vi "Main.vi"() -> ()   [LabVIEW 2020]
doc: "Use this template to build a simple state machine design pattern. Each state executes code and determines which state to transition to."
uses:
  Trigger Cluster.ctl
  TrigSource.ctl
  TrigLevel.ctl
  TrigSpeedCluster.ctl
  controls/State.ctl
  controls/Data.ctl
  MuessageCluster.ctl
  <vilib>/Utility/miscctls.llb/LVRangeTypeDef.ctl
  <vilib>/Utility/sysdir.llb/System Directory Type.ctl
  <vilib>/DAQmx/read.llb/DAQmx Read (Analog 1D Wfm NChan NSamp).vi
  <vilib>/DAQmx/read.llb/DAQmx Read (Counter 2D DBL NChan NSamp).vi
  <vilib>/DAQmx/miscellaneous.llb/DAQmx Fill In Error Info.vi
  <vilib>/measure/mamon.llb/Trigger Detection for 1 Channel.vi
  <vilib>/measure/NI_MAPro.lvlib
panel:
  in  "ManualTrigger":bool caption="Manual Record"
  in  "TrigSpeeds":T1 caption="Record Start/Stop Speeds" {"EndSpeed" min=0 max=12 step=0.1 format="%.1g"; "StartSpeed" min=0 max=12 step=0.1 format="%.1g"}
  in  "TrigCluster":T2={"TrigSource"=enum."Stop Key", "TrigLevel"=enum."Falling"} caption="Trigger Settings"
  out "Loop Time":i32
  out "StopButton":bool
  out "Recording":bool
  out "Trigger":bool
  out "PreTrigger":bool
  out "MPH":dbl format="%.1g"
  in  "Header Row Title":string
  out "Speed Chart":dbl(graph)
  in  "Exit":bool
  # "Treadmill Speed"
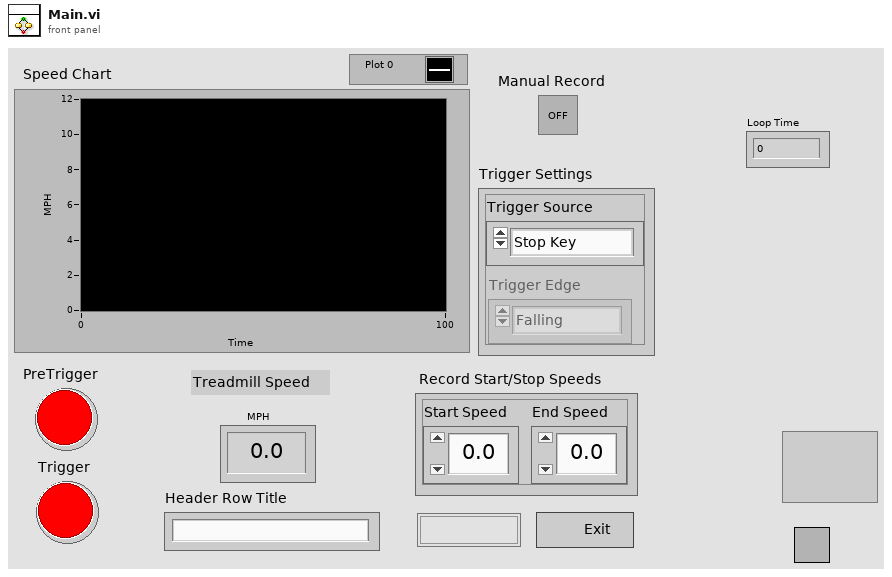
[diagram p1: front panel]
types:
  T1 = typedef "TrigSpeedCluster.ctl" = cluster{"StartSpeed":sgl, "EndSpeed":sgl}
  T2 = typedef "Trigger Cluster.ctl" = cluster{"TrigSource":T3, "TrigLevel":T4}
  T3 = typedef "TrigSource.ctl" = enum16{"Error Condition", "Machine Ctrl (Phase C)", "E-Stop Key", "Stop Key", "Blackout", "Manual"}
  T4 = typedef "TrigLevel.ctl" = enum16{"Falling", "Rising"}
  T5 = typedef "MuessageCluster.ctl" = cluster{"Message":enum16{"Init", "StopRFQ", "Stop", "UserEvent"}, "Message Data":variant}
  T6 = typedef "Data.ctl" = cluster{"Speed Data":dbl, "StopButtonState":bool, "Recording":bool, "PreTrigStateCount":u32, "HeaderString":string, "SpeedTask":refnum<k21>, "AnalogTrigTask":refnum<k21>, "TriggerLevel Data":waveform(dbl)[], "PreTrigTimer(s)":dbl, "MillisecondTimerValue":dbl, "RecordedData":dbl[][], "StopButton":bool, "TrigCluster":T2, "PreTrigState":bool, "TriggerState":bool, "TrigTimeStamp":dbl[], "TrigSpeeds":T1, "ResetTrig?":bool, "SpeedData":dbl[][], "ManualTrigger":bool}
  T7 = typedef "State.ctl" = enum16{"Initialize", "Start Tasks", "Acquire", "Check Trigger", "Check TriggerOrg", "Check for User Event", "StopRFQ", "Update UI", "CheckPreTrigState", "CheckPreTrigStateOrg", "Save MPH/Time Data", "Save Data to CSV", "Restart", "StreamingData", "Exit"}
  T8 = enum8{"Enabled", "Disabled", "Disabled and Grayed Out"}
  T9 = typedef "LVRangeTypeDef.ctl" = cluster{"Minimum":dbl, "Maximum":dbl, "Increment":dbl, "Minor Increment":dbl, "Start":dbl}
  T10 = typedef "System Directory Type.ctl" = i32
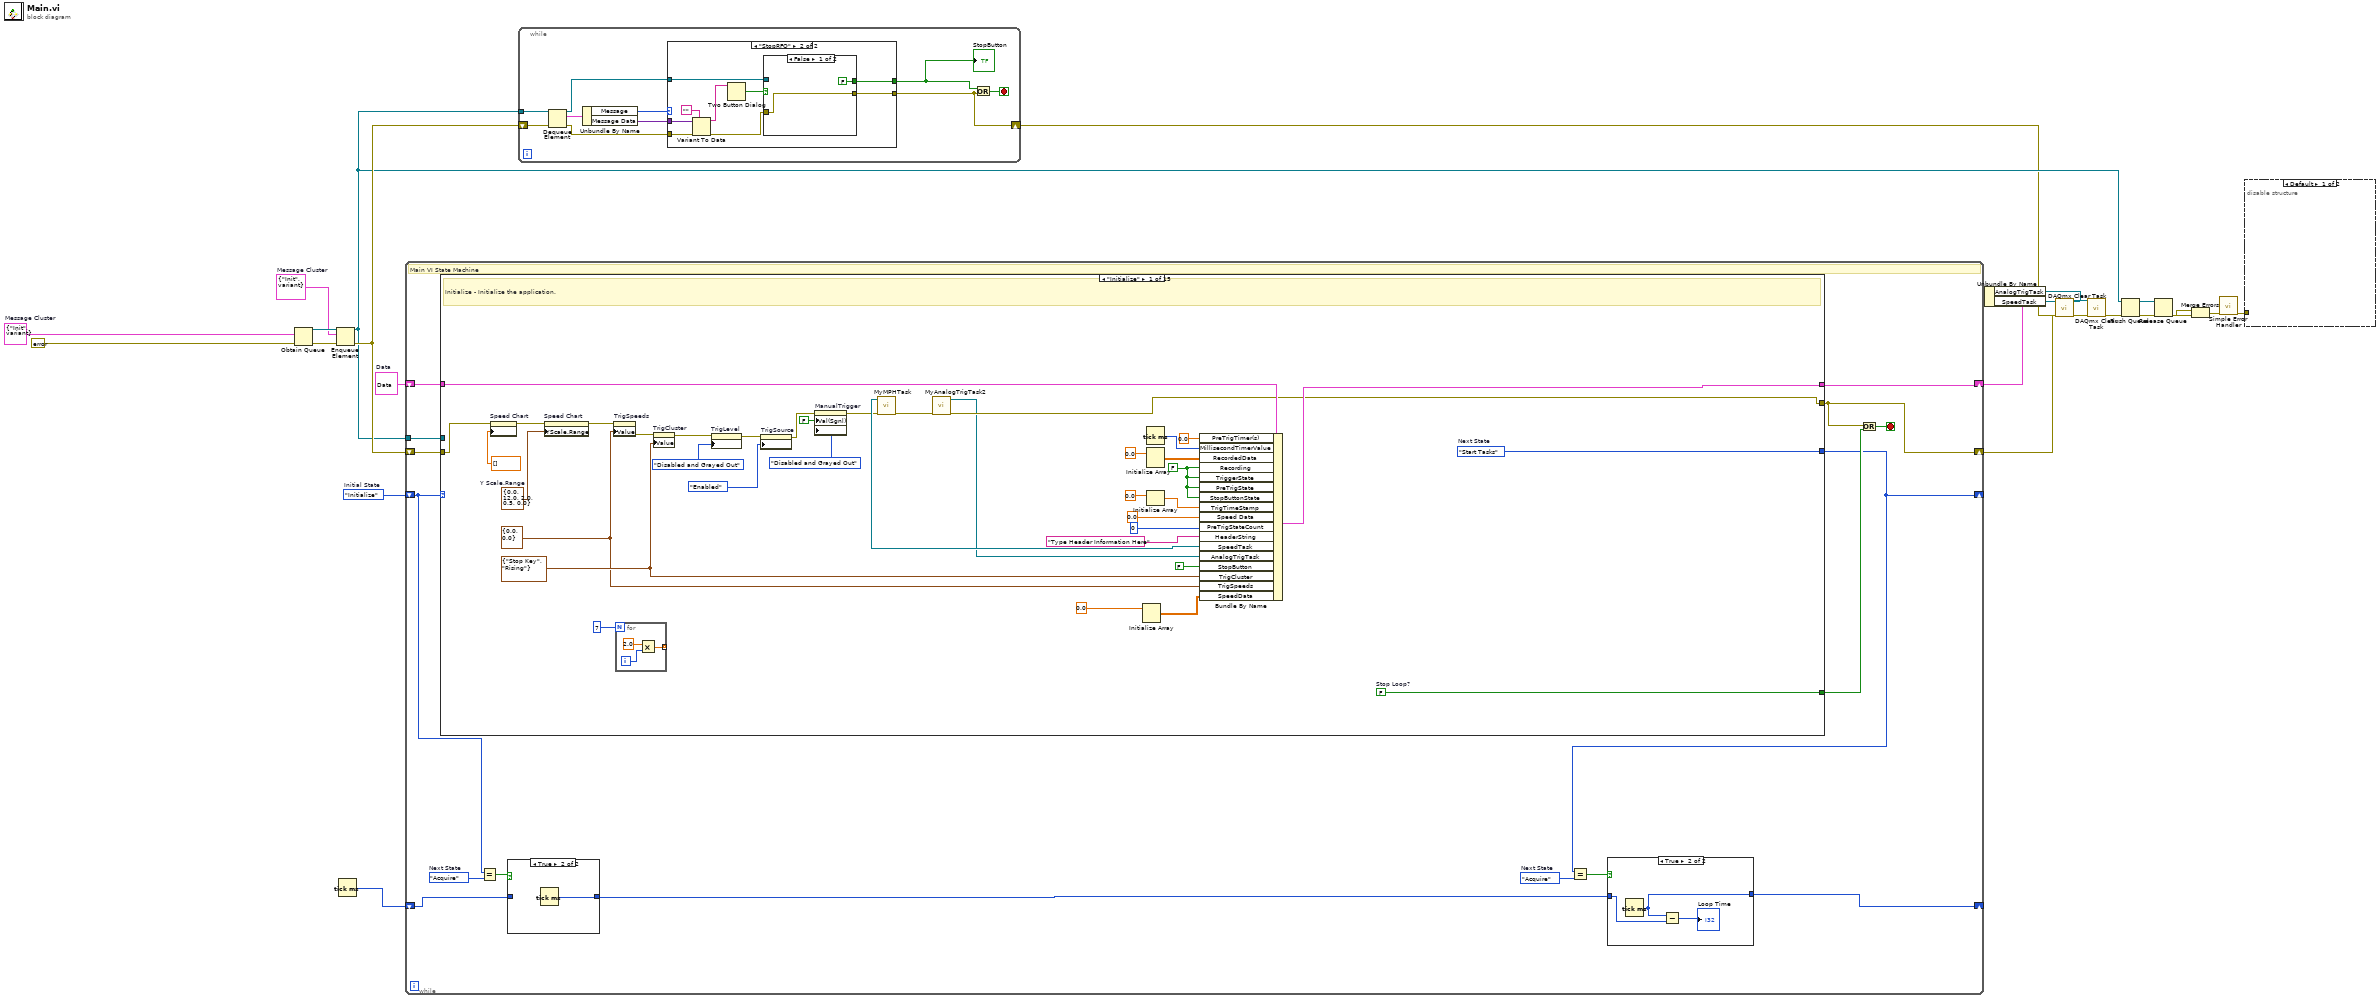
[diagram p0: block diagram]
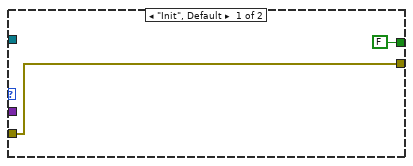
[diagram p2: hidden frame]
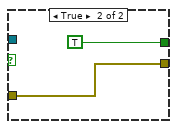
[diagram p3: hidden frame]
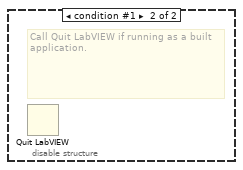
[diagram p4: hidden frame]
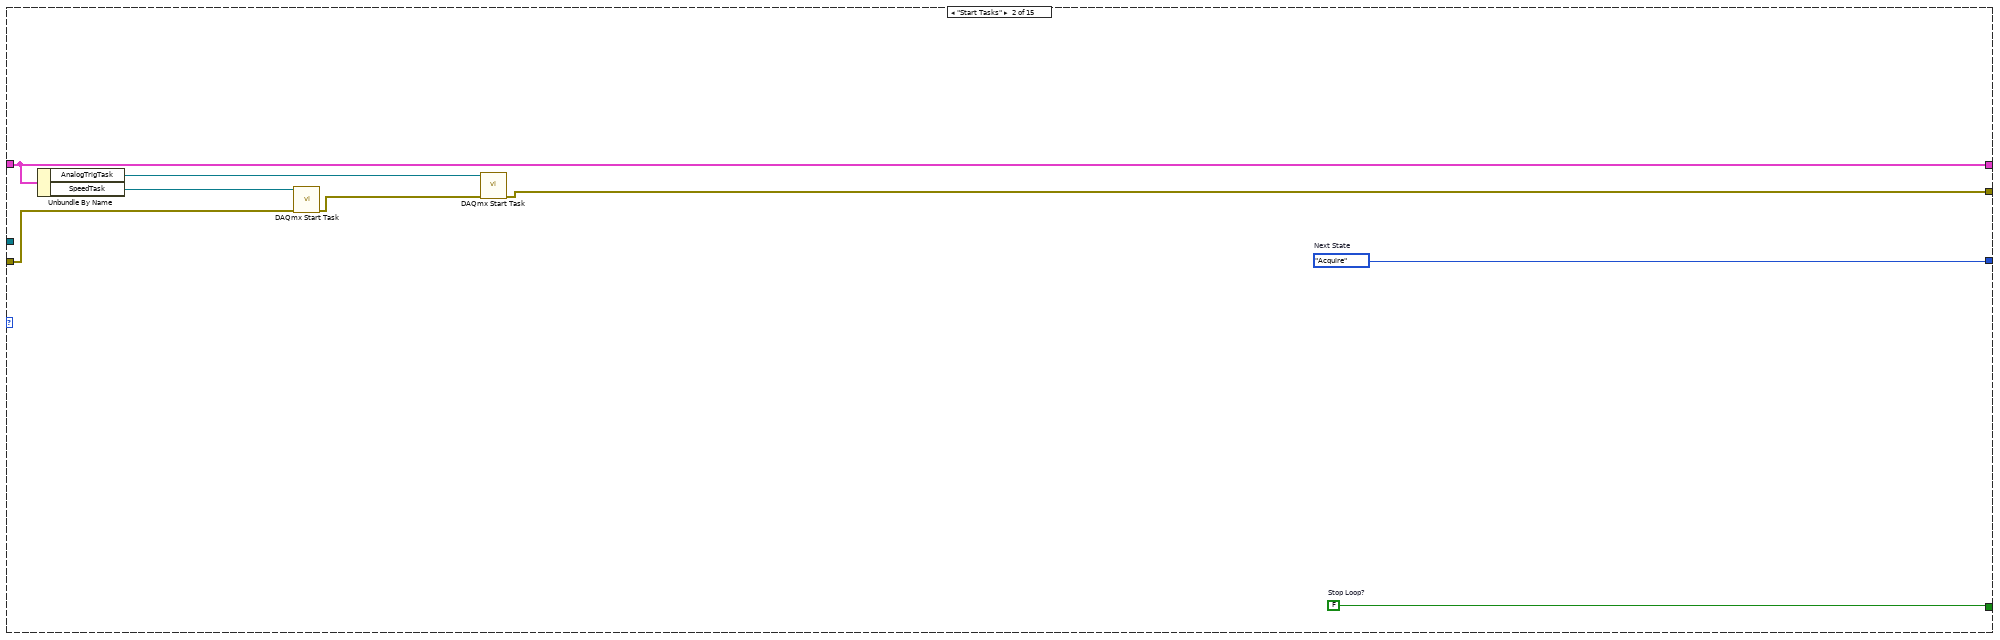
[diagram p7: hidden frame]
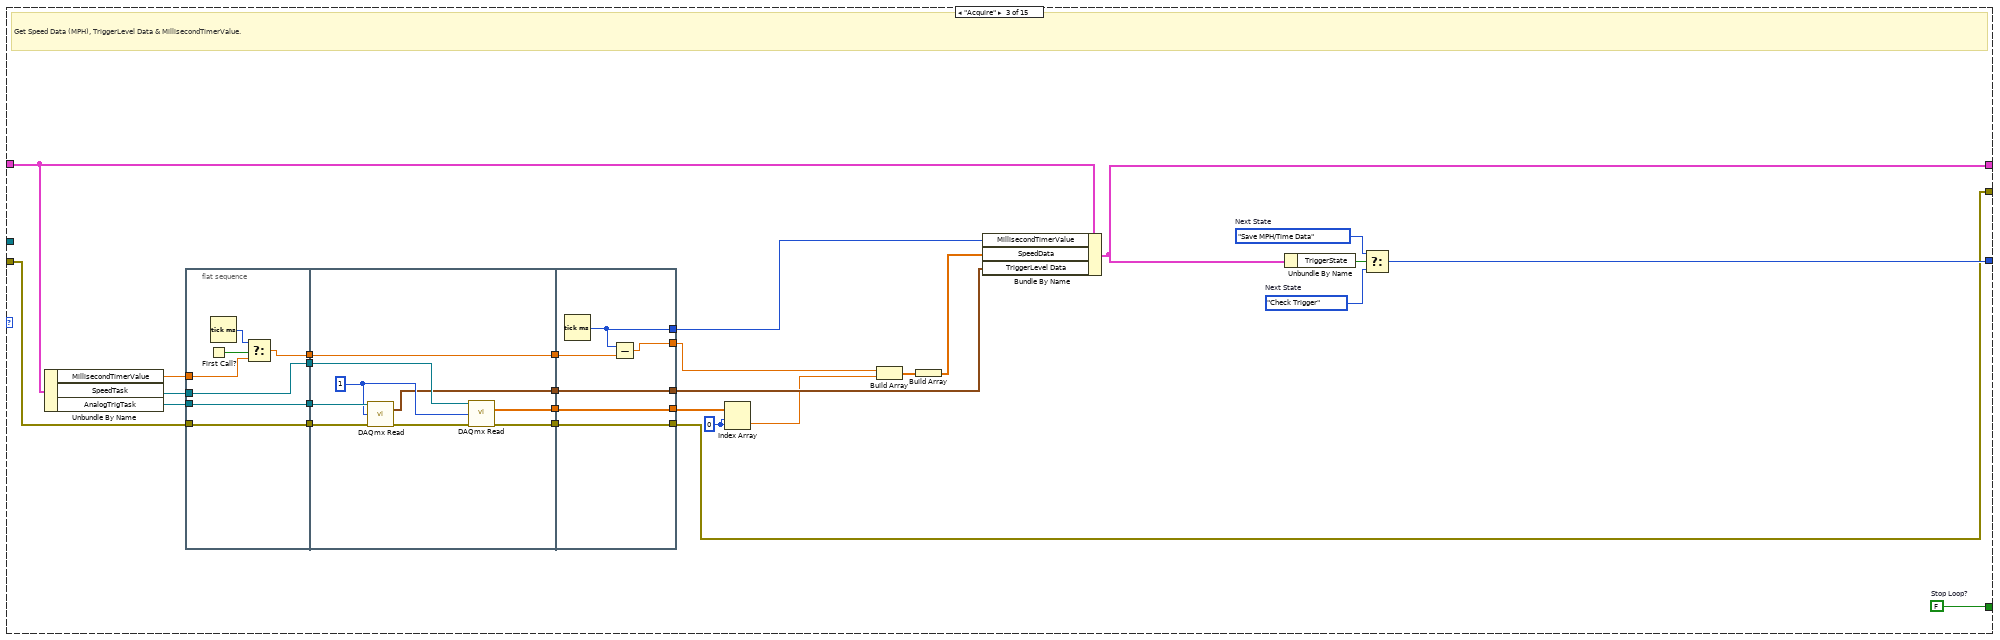
[diagram p8: hidden frame]
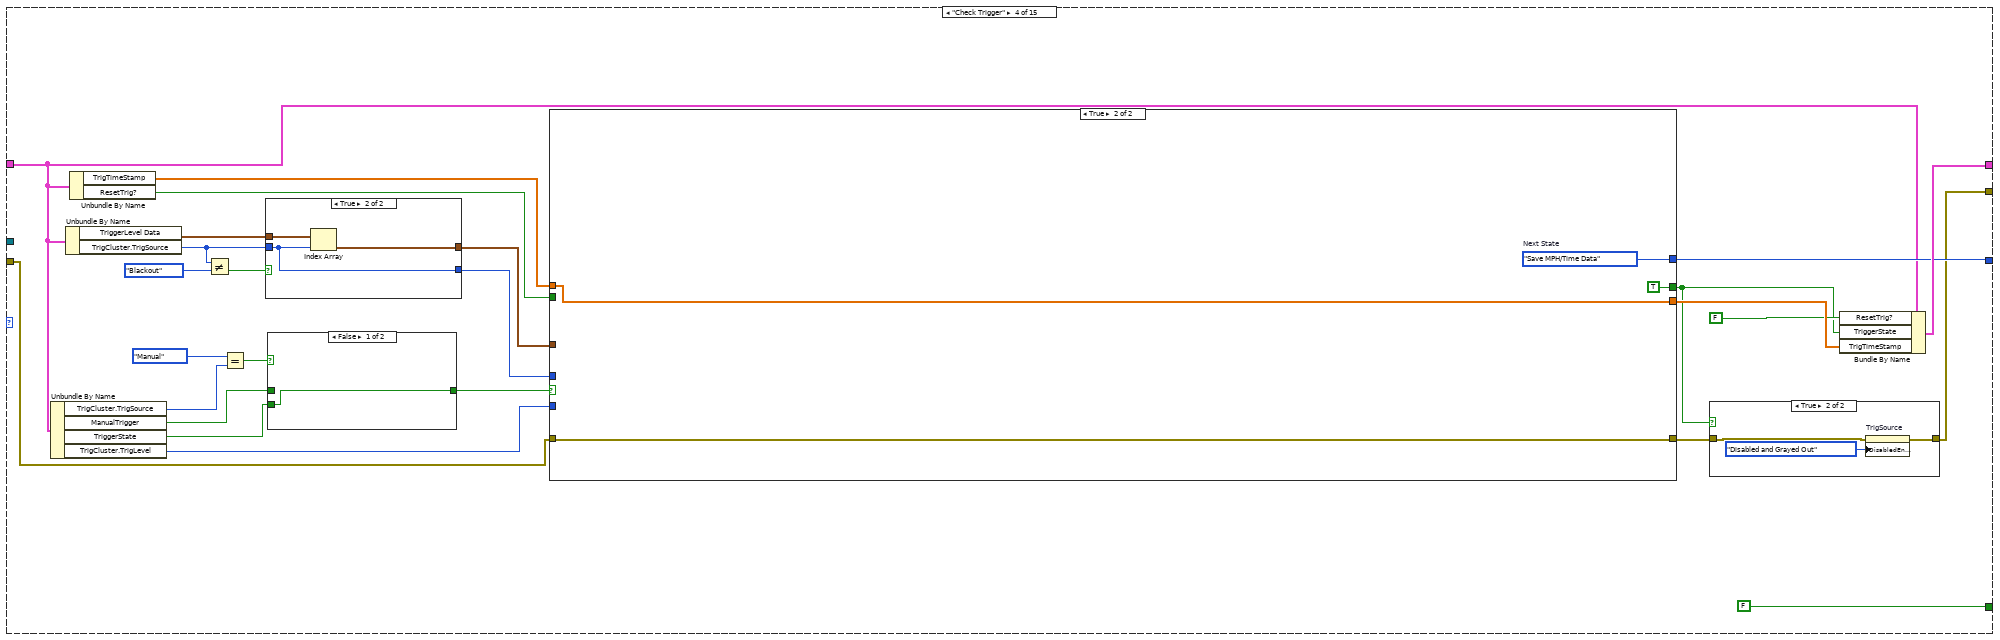
[diagram p9: hidden frame]
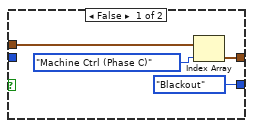
[diagram p12: hidden frame]
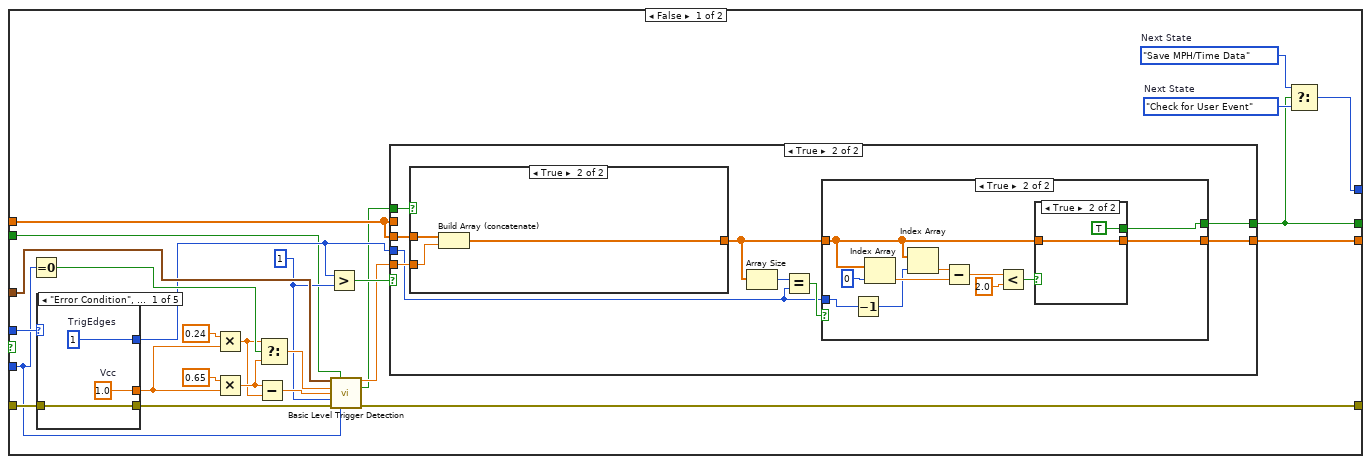
[diagram p13: hidden frame]
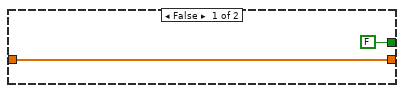
[diagram p15: hidden frame]
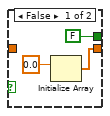
[diagram p16: hidden frame]
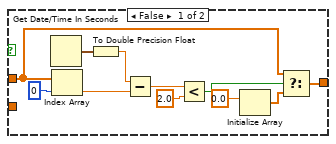
[diagram p17: hidden frame]
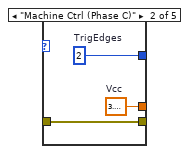
[diagram p18: hidden frame]
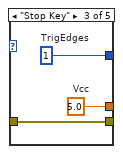
[diagram p19: hidden frame]
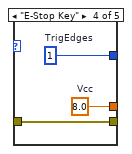
[diagram p20: hidden frame]
diagram:
  w15 = T5 {"Message"=enum."Init", "Message Data"=variant}  # Message Cluster
  w18 = T5 {"Message"=enum."Init", "Message Data"=variant}  # Message Cluster
  w22 = T6 {"Speed Data"=0.0, "StopButtonState"=FALSE, "Recording"=FALSE, "PreTrigStateCount"=0, "HeaderString"="", "SpeedTask"="", "AnalogTrigTask"="", "TriggerLevel Data"=[], "PreTrigTimer(s)"=0.0, "MillisecondTimerValue"=0.0, "RecordedData"=[], "StopButton"=FALSE, "TrigCluster"={"TrigSource"=enum."Stop Key", "TrigLevel"=enum."Falling"}, "PreTrigState"=FALSE, "TriggerState"=FALSE, "TrigTimeStamp"=[], "TrigSpeeds"={"StartSpeed"=0.0, "EndSpeed"=0.0}, "ResetTrig?"=FALSE, "SpeedData"=[], "ManualTrigger"=FALSE}  # Data
  w20 = State."Initialize"  # Initial State
  n1 = Obtain Queue(element data type=w18, error in (no error)=errorcluster {"status"=FALSE, "code"=0, "source"=""} ("error constant")) -> (queue out=w19:refnum<queue>, error out=w17:errorcluster)  [unwired: 3 in, 1 out]
  n2 = Enqueue Element(queue=w19, element=w15, error in (no error)=w17) -> (queue out=w5:refnum<queue>, error out=w14:errorcluster)  [unwired: 1 in, 1 out]
  n3 = Tick Count (ms)() -> (millisecond timer value=w1:u32)
  n4 = while {
    shift-right: [w31] -> _
    shift-left: w20 -> [w27]
    shift-right: [w37] -> w7
    shift-left: w22 -> [w38]
    shift-right: [w33] -> w6
    shift-left: w14 -> [w36]
    tunnel: w5 -> [w32]
    shift-right: [w23] -> _
    shift-left: w1 -> [w25]
    stop <- w34 stop-if-true
    w28 = State."Acquire"  # Next State
    w30 = State."Acquire"  # Next State
    # "Main VI State Machine"
    n5 = case shown="\"Initialize\"" w27 {
      tunnel: [w74 w87 w114 w166 w274 w363 w385 w395 w443 w522 w551 w575 State."Exit" ("Next State") w593 w642] -> w31
      tunnel: [w82 w86 w120 FALSE ("Stop Loop?") w276 w371 w381 w394 w478 w521 w550 w579 w584 w592 w641] -> w35
      tunnel: w38 -> [w81 w93 w108 w152 w271 w372 w384 w393 w481 w539 w568 w580 w582 w591 w645]
      tunnel: [w80 w93 w118 w167 w272 w372 w384 w396 w472 w539 w568 w578 w582 w594 w643] -> w37
      tunnel: w36 -> [w76 w92 w119 w165 w270 w369 _ w397 w471 w516 w545 w571 w581 w587 w646]
      tunnel: [w64 w88 w106 w159 w273 w364 w382 w390 w447 w523 w552 w569 w581 w586 w646] -> w33
      tunnel: w32 -> [_ _ _ _ _ w370 _ _ _ _ _ _ _ _ _]
      frame "Initialize" {
        w57 = T2 {"TrigSource"=enum."Stop Key", "TrigLevel"=enum."Rising"} ("TrigCluster")
        w56 = T1 {"StartSpeed"=0.0, "EndSpeed"=0.0} ("TrigSpeeds")
        w60 = T9 {"Minimum"=0.0, "Maximum"=12.0, "Increment"=2.0, "Minor Increment"=0.5, "Start"=0.0}  # Y Scale.Range
        w74 = State."Start Tasks"  # Next State
        w49 = FALSE ("Replace_Me_Boolean")
        w82 = FALSE  # Stop Loop?
        # "Initialize - Initialize the application."
        n6 = property on="Speed Chart" class="WFChart (strict)"(error in=w76, "History Data"=dbl[] []) -> (error out=w66:errorcluster)  [unwired: 1 in, 1 out]
        n7 = property on="Speed Chart" class="WFChart (strict)"(error in=w66, "YScale.Range"=w60) -> (error out=w59:errorcluster)  [unwired: 1 in, 1 out]
        n8 = property on="TrigSpeeds" class="Clust (strict)"(error in=w59, "Value"=w56) -> (error out=w58:errorcluster)  [unwired: 1 in, 1 out]
        n9 = for {
          N: 7 -> [_]
          tunnel: [w83] -> _ mode=indexing
          i -> [w84]
          n10 = Multiply(x=2.0 ("Speed Data"), y=w84) -> (x*y=w83:dbl)
        }
        n11 = property on="TrigCluster" class="Clust (strict)"(error in=w58, "Value"=w57) -> (error out=w55:errorcluster)  [unwired: 1 in, 1 out]
        n12 = property on="TrigLevel" class="Enum (strict)"(error in=w55, "DisabledEnum"=T8."Disabled and Grayed Out" ("Disabled")) -> (error out=w51:errorcluster)  [unwired: 1 in, 1 out]
        n13 = property on="TrigSource" class="Enum (strict)"(error in=w51, "DisabledEnum"=T8."Enabled" ("Disabled")) -> (error out=w48:errorcluster)  [unwired: 1 in, 1 out]
        n14 = property on="ManualTrigger" class="Bool (strict)"(error in=w48, "Val(Sgnl)"=FALSE ("Value (Signaling)"), "DisabledEnum"=T8."Disabled and Grayed Out" ("Disabled")) -> (error out=w47:errorcluster)  [unwired: 1 in, 1 out]
        n15 = call "MyMPHTask.vi"("error in"=w47) -> ("error out"=w65:errorcluster, "task out"=w75:refnum<k21>)  [unwired: 9 in]
        n16 = call "MyAnalogTrigTask2.vi"("error in"=w65) -> ("error out"=w64:errorcluster, "task out"=w63:refnum<k21>)  [unwired: 9 in]
        n17 = Initialize Array(0.0 ("element")) -> (w53:dbl[][])  [unwired: 2 in]
        n18 = Tick Count (ms)() -> (millisecond timer value=w69:u32)
        n19 = Initialize Array(0.0 ("element")) -> (w72:dbl[][])  [unwired: 2 in]
        n20 = Initialize Array(0.0 ("element")) -> (w62:dbl[])  [unwired: 1 in]
        n21 = Bundle By Name(cluster=w81, "PreTrigTimer(s)"=0.0 ("MillisecondTimerValue"), "MillisecondTimerValue"=w69, "RecordedData"=w72, "Recording"=w49, "TriggerState"=w49, "PreTrigState"=w49, "StopButtonState"=w49, "TrigTimeStamp"=w62, "Speed Data"=0.0, "PreTrigStateCount"=u32 0, "HeaderString"="Type Header Information Here", "SpeedTask"=w75, "AnalogTrigTask"=w63, "StopButton"=FALSE, "TrigCluster"=w57, "TrigSpeeds"=w56, "SpeedData"=w53) -> (w80:T6)
      }
      frame "Start Tasks" {
        w86 = FALSE  # Stop Loop?
        w87 = State."Acquire"  # Next State
        n22 = Unbundle By Name(w93) -> ("AnalogTrigTask"=w89:refnum<k21>, "SpeedTask"=w90:refnum<k21>)
        n23 = call <vilib>:"DAQmx Start Task.vi"("task/channels in"=w90, "error in"=w92) -> ("error out"=w91:errorcluster)  [unwired: 12 in, 1 out]
        n24 = call <vilib>:"DAQmx Start Task.vi"("task/channels in"=w89, "error in"=w91) -> ("error out"=w88:errorcluster)  [unwired: 12 in, 1 out]
      }
      frame "Acquire" {
        w116 = State."Save MPH/Time Data"  # Next State
        w120 = FALSE  # Stop Loop?
        w121 = 0 ("index (row)")
        w115 = State."Check Trigger"  # Next State
        # "Get Speed Data (MPH), TriggerLevel Data & MillisecondTimerValue."
        n25 = Unbundle By Name(w108) -> ("MillisecondTimerValue"=w99:dbl, "SpeedTask"=w111:refnum<k21>, "AnalogTrigTask"=w112:refnum<k21>)
        n26 = flat-sequence {
          tunnel: w111 -> [w126]
          tunnel: w112 -> [w127]
          tunnel: w119 -> [w128]
          tunnel: [w128] -> w102
          tunnel: [w127] -> w101
          tunnel: [w126] -> w100
          tunnel: w99 -> [w124]
          tunnel: [w122] -> w97
          tunnel: [w137] -> w113
          tunnel: [w131] -> w110
          tunnel: [w130] -> w109
          tunnel: w102 -> [w136]
          tunnel: w101 -> [w135]
          tunnel: w100 -> [w134]
          tunnel: [w129] -> w98
          tunnel: w97 -> [w129]
          tunnel: [w143] -> w106
          tunnel: w113 -> [w143]
          tunnel: [w142] -> w95
          tunnel: w110 -> [w142]
          tunnel: [w141] -> w107
          tunnel: w109 -> [w141]
          tunnel: [w140] -> w105
          tunnel: w98 -> [w139]
          tunnel: [w138] -> w96
          frame #0 {
            n27 = First Call?() -> (First Call?: T/F=w125:bool)
            n28 = Tick Count (ms)() -> (millisecond timer value=w123:u32)
            n29 = Select(t=w123, s=w125, f=w124) -> (s? t:f=w122:dbl)
          }
          frame #1 {
            w133 = 1 ("number of samples per channel")
            n30 = call-poly <vilib>:"DAQmx Read.vi"("task/channels in"=w135, "number of samples per channel"=w133, "error in"=w136) -> ("data"=w130:waveform(dbl)[], "error out"=w132:errorcluster)  [unwired: 10 in, 1 out]
            n31 = call-poly <vilib>:"DAQmx Read.vi"("task/channels in"=w134, "number of samples per channel"=w133, "error in"=w132) -> ("data"=w131:dbl[][], "error out"=w137:errorcluster)  [unwired: 10 in, 1 out]
          }
          frame #2 {
            n32 = Tick Count (ms)() -> (millisecond timer value=w138:u32)
            n33 = Subtract(x=w138, y=w139) -> (x-y=w140:dbl)
          }
        }
        n34 = Index Array(array=w95, index (row)=w121, index (col)=w121) -> (element=w94:dbl)
        n35 = Build Array(w105, w94) -> (w104:dbl[])
        n36 = Build Array(w104) -> (w103:dbl[][])
        n37 = Bundle By Name(cluster=w108, "MillisecondTimerValue"=w96, "SpeedData"=w103, "TriggerLevel Data"=w107) -> (w118:T6)
        n38 = Unbundle By Name(w118) -> ("TriggerState"=w117:bool)
        n39 = Select(t=w116, s=w117, f=w115) -> (s? t:f=w114:T7)
      }
      frame "Check Trigger" {
        n40 = Unbundle By Name(w152) -> ("TrigCluster.TrigSource"=w148:T3, "ManualTrigger"=w145:bool, "TriggerState"=w144:bool, "TrigCluster.TrigLevel"=w153:T4)
        n41 = Unbundle By Name(w152) -> ("TriggerLevel Data"=w156:waveform(dbl)[], "TrigCluster.TrigSource"=w155:T3)
        n42 = Unbundle By Name(w152) -> ("TrigTimeStamp"=w158:dbl[], "ResetTrig?"=w157:bool)
        n43 = Not Equal?(x=w155, y=TrigSource."Blackout" ("TrigCluster.TrigSource")) -> (x != y?=w150:bool)
        n44 = Equal?(x=TrigSource."Manual", y=w148) -> (x = y?=w149:bool)
        n45 = case shown="True" w150 {
          tunnel: w156 -> [w178 w181]
          tunnel: w155 -> [_ w179]
          tunnel: [w176 w180] -> w163
          tunnel: [TrigSource."Blackout" ("TrigCluster.TrigSource") w179] -> w162
          frame False {
            n46 = Index Array(array=w178, index=TrigSource."Machine Ctrl (Phase C)" ("TrigCluster.TrigSource")) -> (element=w176:waveform(dbl))
          }
          frame True {
            n47 = Index Array(array=w181, index=w179) -> (element=w180:waveform(dbl))
          }
        }
        n48 = case shown="False" w149 {
          tunnel: [w169 w170] -> w146
          tunnel: w145 -> [_ w170]
          tunnel: w144 -> [w169 _]
          frame False {
          }
          frame True {
          }
        }
        n49 = case shown="True" w146 {
          tunnel: w153 -> [w183 _]
          tunnel: [w193 TRUE] -> w151
          tunnel: [w205 w269] -> w166
          tunnel: w163 -> [w197 _]
          tunnel: w165 -> [w187 w267]
          tunnel: w158 -> [w192 w266]
          tunnel: [w194 w266] -> w164
          tunnel: [w195 w267] -> w160
          tunnel: w162 -> [w185 _]
          tunnel: w157 -> [w184 _]
          frame False {
            w188 = 1 ("y")
            w207 = State."Save MPH/Time Data"  # Next State
            w206 = State."Check for User Event"  # Next State
            n50 = Equal To 0?(x=w183) -> (x = 0?=w201:bool)
            n51 = case shown="\"Error Condition\", Default" w185 {
              tunnel: [w253 w256 w259 w262 w265] -> w202
              tunnel: [w252 w255 w258 w261 w264] -> w189
              tunnel: w187 -> [w251 w254 w257 w260 w263]
              tunnel: [w251 w254 w257 w260 w263] -> w186
              frame "Error Condition", Default {
                w252 = 1  # TrigEdges
                w253 = sgl 1.0  # Vcc
              }
              frame "Machine Ctrl (Phase C)" {
                w255 = 2  # TrigEdges
                w256 = sgl 3.3  # Vcc
              }
              frame "Stop Key" {
                w258 = 1  # TrigEdges
                w259 = sgl 5.0  # Vcc
              }
              frame "E-Stop Key" {
                w261 = 1  # TrigEdges
                w262 = sgl 8.0  # Vcc
              }
              frame "Blackout" {
                w264 = 1  # TrigEdges
                w265 = sgl 5.0  # Vcc
              }
            }
            n52 = Multiply(x=0.24, y=w202) -> (x*y=w199:dbl)
            n53 = Multiply(x=0.65, y=w202) -> (x*y=w200:dbl)
            n54 = Subtract(x=w200, y=w199) -> (x-y=w190:dbl)
            n55 = Select(t=w199, s=w201, f=w200) -> (s? t:f=w198:dbl)
            n56 = Greater?(x=w189, y=w188) -> (0:w196:bool)
            n57 = call-poly <vilib>:"Basic Level Trigger Detection.vi"("signal in"=w197, "reset"=w184, "level"=w198, "hysteresis"=w190, "location mode"=w188, "error in (no error)"=w186, "trigger slope"=w183) -> ("trigger location"=w191:dbl, "trigger detected?"=w182:bool, "error out"=w195:errorcluster)  [unwired: 6 in]
            n58 = case shown="True" w196 {
              tunnel: [w209 w211] -> w193
              tunnel: w182 -> [w209 w218]
              tunnel: w192 -> [w208 _]
              tunnel: [w208 w210] -> w194
              tunnel: w189 -> [_ w212]
              tunnel: w192 -> [_ w217]
              tunnel: w191 -> [_ w216]
              frame False {
              }
              frame True {
                n59 = case shown="True" w218 {
                  tunnel: w217 -> [w240 w250]
                  tunnel: w216 -> [_ w249]
                  tunnel: [w237 w248] -> w213
                  frame False {
                    n60 = Get Date/Time In Seconds() -> (seconds since 1Jan1904=w245:timestamp)
                    n61 = Index Array(array=w240, index=0) -> (element=w243:dbl)
                    n62 = To Double Precision Float(number=w245) -> (double precision float=w246:dbl)
                    n63 = Subtract(x=w246, y=w243) -> (x-y=w247:dbl)
                    n64 = Less?(x=w247, y=2.0) -> (x < y?=w241:bool)
                    n65 = Initialize Array(0.0 ("element")) -> (w238:dbl[])  [unwired: 1 in]
                    n66 = Select(t=w240, s=w241, f=w238) -> (s? t:f=w237:dbl[])
                  }
                  frame True {
                    n67 = Build Array (concatenate)(w250, w249) -> (w248:dbl[])
                  }
                }
                n68 = Array Size(array=w213) -> (size(s)=w215:i32)
                n69 = Equal?(x=w215, y=w212) -> (x = y?=w214:bool)
                n70 = case shown="True" w214 {
                  tunnel: w213 -> [w220 w226]
                  tunnel: [w220 w225] -> w210
                  tunnel: [FALSE w224] -> w211
                  tunnel: w212 -> [_ w222]
                  frame False {
                  }
                  frame True {
                    n71 = Decrement(x=w222) -> (x-1=w223:i32)
                    n72 = Index Array(array=w226, index=0) -> (element=w229:dbl)
                    n73 = Index Array(array=w226, index=w223) -> (element=w230:dbl)
                    n74 = Subtract(x=w230, y=w229) -> (x-y=w228:dbl)
                    n75 = Less?(x=w228, y=2.0) -> (x < y?=w227:bool)
                    n76 = case shown="True" w227 {
                      tunnel: w226 -> [_ w236]
                      tunnel: [w233 w236] -> w225
                      tunnel: [FALSE TRUE] -> w224
                      frame False {
                        n77 = Initialize Array(0.0 ("element")) -> (w233:dbl[])  [unwired: 1 in]
                      }
                      frame True {
                      }
                    }
                  }
                }
              }
            }
            n78 = Select(t=w207, s=w193, f=w206) -> (s? t:f=w205:T7)
          }
          frame True {
            w269 = State."Save MPH/Time Data"  # Next State
          }
        }
        n79 = case shown="True" w151 {
          tunnel: w160 -> [w171 w174]
          tunnel: [w171 w173] -> w159
          frame False {
          }
          frame True {
            n80 = property on="TrigSource" class="Enum (strict)"(error in=w174, "DisabledEnum"=T8."Disabled and Grayed Out" ("Disabled")) -> (error out=w173:errorcluster)  [unwired: 1 in, 1 out]
          }
        }
        n81 = Bundle By Name(cluster=w152, "ResetTrig?"=FALSE, "TriggerState"=w151, "TrigTimeStamp"=w164) -> (w167:T6)
      }
      frame "Check for User Event" {
        w276 = FALSE  # Stop Loop?
        # "Wait for Event - Use an Event Structure to monitor the user interface for events that run different states of the state machine."
        n82 = event shown="[3] \"ManualTrigger\": Value Change" {
          selector: _ -> [_ _ _ _ _ _]
          dyn-events: _ -> [_ _ _ _ _ _]
          timeout: 1 -> [_ _ _ _ _ _]
          tunnel: [w279 w299 w312 State."Update UI" ("Next State") w325 w360] -> w274
          tunnel: w271 -> [w278 w298 w310 w321 w327 w361]
          tunnel: [w278 w297 w309 w320 w326 w361] -> w272
          tunnel: w270 -> [w277 w292 w311 w318 w328 w362]
          tunnel: [w277 w291 w311 w317 w324 w362] -> w273
          event "Exit": Value Change {
            w279 = State."StopRFQ"  # Next State
            n83 = event-data() -> ()  [unwired: 1 in, 1 out]
          }
          event Value Change {
            w299 = State."Update UI"  # Next State
            n84 = event-data() -> ()  [unwired: 1 in, 6 out]
            n85 = Unbundle By Name("TrigCluster") -> ("TrigSource"=w289:T3)  [unwired: 1 out]
            n86 = Equal?(x=w289, y=TrigSource."Blackout" ("TrigSource")) -> (x = y?=w294:bool)
            n87 = case shown="False" w294 {
              tunnel: w292 -> [w301 w304]
              tunnel: [w302 w303] -> w287
              frame False {
                n88 = property on="TrigLevel" class="Enum (strict)"(error in=w301, "Value"=TrigLevel."Rising") -> (error out=w302:errorcluster)  [unwired: 1 in, 1 out]
              }
              frame True {
                n89 = property on="TrigLevel" class="Enum (strict)"(error in=w304, "Value"=TrigLevel."Falling") -> (error out=w303:errorcluster)  [unwired: 1 in, 1 out]
              }
            }
            n90 = Equal?(x=w289, y=TrigSource."Manual") -> (x = y?=w284:bool)
            n91 = Select(t=0.0, s=w284, f=2.0) -> (s? t:f=w285:dbl)
            n92 = property on="ManualTrigger" class="Bool (strict)"(error in=w287, "DisabledEnum"=w285, "Val(Sgnl)"=FALSE ("Value (Signaling)")) -> (error out=w286:errorcluster)  [unwired: 1 in, 1 out]
            n93 = property on="TrigLevel" class="Enum (strict)"(error in=w286) -> (error out=w291:errorcluster, "Value"=w290:T4)  [unwired: 1 in, 1 out]
            n94 = Bundle By Name(cluster=w298, "TrigCluster.TrigSource"=w289, "ManualTrigger"=FALSE, "TrigCluster.TrigLevel"=w290, "ResetTrig?"=TRUE) -> (w297:T6)
          }
          event Value Change {
            w312 = State."Update UI"  # Next State
            n95 = event-data() -> ()  [unwired: 1 in, 6 out]
            n96 = Unbundle By Name("TrigSpeeds") -> ("StartSpeed"=w307:sgl, "EndSpeed"=w306:sgl)
            n97 = Bundle By Name(cluster=w310, "TrigSpeeds.StartSpeed"=w307, "TrigSpeeds.EndSpeed"=w306) -> (w309:T6)
          }
          event "ManualTrigger": Value Change {
            n98 = event-data() -> ()  [unwired: 1 in, 6 out]
            n99 = Select(t=2.0, s="ManualTrigger", f=0.0) -> (s? t:f=w316:dbl)
            n100 = Bundle By Name(cluster=w321, "ManualTrigger"="ManualTrigger") -> (w320:T6)
            n101 = property on="TrigCluster" class="Clust (strict)"(error in=w318, "DisabledEnum"=w316) -> (error out=w317:errorcluster)  [unwired: 1 in, 1 out]
          }
          event "Header Row Title": Value Change {
            w325 = State."Update UI"  # Next State
            n102 = event-data() -> ()  [unwired: 1 in, 1 out]
            n103 = Empty String/Path?(string/path="Header Row Title") -> (empty?=w322:bool)
            n104 = case shown="False" w322 {
              tunnel: "Header Row Title" -> [w337 w353]
              tunnel: w328 -> [w336 w355]
              tunnel: w327 -> [w332 w356]
              tunnel: [w331 w354] -> w326
              tunnel: [w329 w355] -> w324
              frame False {
                n105 = call "CheckFileName.vi"("error in"=w336, "Path String"=w337) -> ("error out"=w330:errorcluster, "Offset to Bad Character(s)"=w334:i32[], "Bad Filename?"=w335:bool, "Path String Out"=w333:string)  [unwired: 5 in, 1 out]
                n106 = case shown="True" w335 {
                  tunnel: w334 -> [_ w346]
                  tunnel: w333 -> [w340 w345]
                  tunnel: w332 -> [w341 w344]
                  tunnel: [w339 w343] -> w331
                  tunnel: w330 -> [w338 w342]
                  tunnel: [w338 w342] -> w329
                  frame False {
                    n107 = Bundle By Name(cluster=w341, "HeaderString"=w340) -> (w339:T6)
                  }
                  frame True {
                    n108 = for {
                      tunnel: w346 -> [w350] mode=indexing
                      tunnel: w345 -> [w352]
                      tunnel: w344 -> [w349]
                      tunnel: [w347] -> w343
                      n109 = Replace Substring(2:1 ("length (len. of substring)"), 3:w350, 5:w352) -> (1:w348:string)  [unwired: 1 in, 1 out]
                      n110 = Bundle By Name(cluster=w349, "HeaderString"=w348) -> (w347:T6)
                    }
                  }
                }
              }
              frame True {
                n111 = Bundle By Name(cluster=w356, "HeaderString"=w353) -> (w354:T6)
              }
            }
          }
          event Timeout {
            w357 = State."Update UI"  # Next State
            w359 = State."Exit"  # Next State
            n112 = event-data() -> ()  [unwired: 1 in, 1 out]
            n113 = local read "StopButton"() -> (w358:bool)
            n114 = Select(t=w359, s=w358, f=w357) -> (s? t:f=w360:T7)
          }
        }
      }
      frame "StopRFQ" {
        w363 = State."Update UI"  # Initial State
        w366 = T5 {"Message"=enum."StopRFQ", "Message Data"=variant}  # Message Cluster
        w371 = FALSE  # Stop Loop?
        n115 = Bundle By Name(cluster=w366, "Message"=enum16{"Init", "StopRFQ", "Stop", "UserEvent"}."StopRFQ", "Message Data"="Are you sure you want to Exit?") -> (w367:T5)
        n116 = Enqueue Element(queue=w370, element=w367, error in (no error)=w369) -> (error out=w364:errorcluster)  [unwired: 1 in, 2 out]
      }
      frame "Update UI" {
        w381 = FALSE  # Stop Loop?
        w379 = T8."Enabled" ("Disabled")
        w380 = T8."Disabled and Grayed Out" ("Disabled")
        w385 = State."Acquire"  # Next State
        n117 = Unbundle By Name(w384) -> ("PreTrigState"=w383:bool, "Recording"=w378:bool)
        n118 = Unbundle By Name(w384) -> ("SpeedData"=w376:dbl[][], "PreTrigState"=→"PreTrigger":bool, "TriggerState"=→"Trigger":bool, "HeaderString"=w387:string, "Recording"=→"Recording":bool)
        n119 = Index Array(array=w376, index (row)=0, index (col)=1 ("disabled index (col)")) -> (element=→"Speed Chart" →"MPH":dbl)
        n120 = local write "Header Row Title"(w387) -> ()
        n121 = Select(t=w380, s=w383, f=w379) -> ()  [unwired: 1 out]
        n122 = Select(t=w380, s=w378, f=w379) -> (s? t:f=w377:T8)
        n123 = property on="Header Row Title" class="Str"("DisabledEnum"=w377) -> (error out=w382:errorcluster)  [unwired: 2 in, 1 out]
      }
      frame "CheckPreTrigState" {
        w394 = FALSE  # Stop Loop?
        n124 = Unbundle By Name(w393) -> ("PreTrigState"=w392:bool, "Speed Data"=w400:dbl, "TrigSpeeds.StartSpeed"=w401:sgl)
        n125 = To Single Precision Float(number=w401) -> (single precision float=w399:sgl)
        n126 = call "CheckSpeedTol (SubVI).vi"("error in (no error)"=w397, "Target Speed"=w399, "Actual Speed"=w400) -> ("error out (no error)"=w391:errorcluster, "Speed in Range?"=w398:bool)  [unwired: 7 in]
        n127 = case shown="False" w392 {
          tunnel: w393 -> [w409 w438]
          tunnel: [w407 w437] -> w396
          tunnel: [w405 w433] -> w395
          tunnel: w398 -> [w406 w436]
          tunnel: w391 -> [w404 w432]
          tunnel: [w402 w432] -> w390
          frame False {
            # "If the previous PreTrigState was false then check to see if the current belt speed meets the minimum speed for a PreTrigState."
            n128 = case shown="True" w406 {
              tunnel: w409 -> [w422 w425]
              tunnel: [w421 w431] -> w408
              tunnel: w404 -> [w417 w427]
              tunnel: [FALSE ("Minimum Dwell Met?") w424] -> w403
              tunnel: [w417 w423] -> w402
              frame False {
                # "Clears the PreTrigState and  timer value if the PreTrigState drops below StartSpeed"
                n129 = Bundle By Name(cluster=w422, "PreTrigState"=FALSE, "PreTrigTimer(s)"=0.0) -> (w421:T6)
              }
              frame True {
                # "Add currentMillisecondTimerValue to the Previous PreTrigTimer count."
                n130 = Unbundle By Name(w425) -> ("PreTrigTimer(s)"=w430:dbl, "MillisecondTimerValue"=w429:dbl)
                n131 = call "ElapsedTimeCounter.vi"("Error In"=w427, "Dwell Time (seconds)"=0.65, "InitialMillisecondTimerValue"=w429, "Elapsed Seconds (In)"=w430) -> ("Error Out"=w423:errorcluster, "Minimum Dwell Met?"=w424:bool, "Elapsed Seconds (Out)"=w426:dbl)  [unwired: 5 in]
                n132 = Bundle By Name(cluster=w425, "PreTrigTimer(s)"=w426) -> (w431:T6)
              }
            }
            n133 = case shown="True" w403 {
              tunnel: w408 -> [w411 w416]
              tunnel: [w411 w415] -> w407
              tunnel: [w410 w413] -> w405
              frame False {
                w410 = State."Check for User Event"  # Next State
              }
              frame True {
                w413 = State."Check Trigger"  # Next State
                # "Set PreTrigState if PreTrigTimer => 0.65 sec."
                n134 = Bundle By Name(cluster=w416, "PreTrigState"=TRUE, "PreTrigTimer(s)"=0.0) -> (w415:T6)
              }
            }
          }
          frame True {
            w434 = State."Check for User Event"  # Next State
            w435 = State."Check Trigger"  # Next State
            # "If PreTrigState True then (Check Trigger)"
            n135 = Bundle By Name(cluster=w438, "PreTrigState"=w436) -> (w437:T6)
            n136 = Select(t=w435, s=w436, f=w434) -> (s? t:f=w433:T7)
          }
        }
      }
      frame "Save MPH/Time Data" {
        w451 = 0 ("index (row)")
        w469 = 0 ("index (row)")
        w478 = FALSE  # Stop Loop?
        n137 = Unbundle By Name(w481) -> ("RecordedData"=w466:dbl[][], "SpeedData"=w450:dbl[][])
        n138 = Array Size(array=w466) -> (size(s)=w474:i32[])
        n139 = Index Array(array=w474, index=0) -> (element=w455:i32)
        n140 = Decrement(x=w455) -> (x-1=w473:i32)
        n141 = Index Array(array=w450, index (row)=0, index (col)=1) -> (element=w461:dbl)
        n142 = Index Array(array=w450, index (row)=w469, index (col)=w469) -> (element=w467:dbl)
        n143 = Index Array(array=w466, index (row)=w473, index (col)=0 ("index (row)")) -> (element=w465:dbl)
        n144 = Divide(x=w467, y=1000.0) -> (x/y=w464:dbl)
        n145 = Add(x=w465, y=w464) -> (x+y=w456:dbl)
        n146 = Equal To 0?(x=w455) -> (x = 0?=w454:bool)
        n147 = Select(t=0.0, s=w454, f=w456) -> (s? t:f=w452:dbl)
        n148 = Build Array(w452, w461) -> (w480:dbl[])
        n149 = Build Array (concatenate)(w466, w480) -> (w479:dbl[][])
        n150 = Bundle By Name(cluster=w481, "RecordedData"=w479, "Recording"=TRUE) -> (w439:T6)
        n151 = Unbundle By Name(w439) -> ("PreTrigTimer(s)"=w448:dbl, "SpeedData"=w457:dbl[][], "TrigSpeeds.EndSpeed"=w470:sgl)
        n152 = Unbundle By Name(w439) -> ("TrigCluster.TrigSource"=w441:T3)
        n153 = Index Array(array=w457, index (row)=w451, index (col)=w451) -> (element=w449:dbl)
        n154 = Index Array(array=w457, index (row)=0, index (col)=1 ("disabled index (col)")) -> (element=w458:dbl)
        n155 = Equal?(x=w441, y=TrigSource."Manual") -> (x = y?=w442:bool)
        n156 = case shown="True" w442 {
          tunnel: w471 -> [w491 w504]
          tunnel: w470 -> [w490 _]
          tunnel: w458 -> [w489 _]
          tunnel: w449 -> [w486 _]
          tunnel: w448 -> [w485 _]
          tunnel: [w484 w504] -> w447
          tunnel: [w483 w502] -> w446
          tunnel: [w482 0.0 ("Elapsed Seconds (Out)")] -> w445
          tunnel: w439 -> [_ w506]
          frame False {
            n157 = call "CheckSpeedTol (SubVI).vi"("error in (no error)"=w491, "Target Speed"=w490, "Actual Speed"=w489) -> ("error out (no error)"=w487:errorcluster, "Speed in Range?"=w488:bool)  [unwired: 7 in]
            n158 = case shown="False" w488 {
              tunnel: w487 -> [w492 w500]
              tunnel: w486 -> [_ w499]
              tunnel: w485 -> [w494 w498]
              tunnel: [w494 w497] -> w482
              tunnel: [w492 w496] -> w484
              tunnel: [FALSE ("Minimum Dwell Met?") w495] -> w483
              frame False {
              }
              frame True {
                n159 = call "ElapsedTimeCounter.vi"("Error In"=w500, "Dwell Time (seconds)"=25.0, "InitialMillisecondTimerValue"=w499, "Elapsed Seconds (In)"=w498) -> ("Error Out"=w496:errorcluster, "Minimum Dwell Met?"=w495:bool, "Elapsed Seconds (Out)"=w497:dbl)  [unwired: 5 in]
              }
            }
          }
          frame True {
            n160 = Unbundle By Name(w506) -> ("ManualTrigger"=w505:bool)
            n161 = Not(x=w505) -> (.not. x?=w502:bool)
          }
        }
        n162 = case shown="False" w446 {
          tunnel: [w508 0.0] -> w444
          tunnel: w445 -> [w508 _]
          tunnel: [w507 w509] -> w443
          frame False {
            w507 = State."Check for User Event"  # Next State
          }
          frame True {
            w509 = State."Save Data to CSV"  # Next State
          }
        }
        n163 = Bundle By Name(cluster=w439, "PreTrigTimer(s)"=w444) -> (w472:T6)
      }
      frame "Save Data to CSV" {
        w521 = FALSE  # Stop Loop?
        w522 = State."Restart"  # Next State
        w530 = T10 2 items=["User Home"=0, "User Desktop"=1, "User Documents"=2, "User Application Data"=3, "User Preferences"=4, "User Temporary"=5, "Public Documents"=6, "Public Application Data"=7, "Public Preferences"=8, "Public Cache"=13, "System Core Libraries"=9, "System Installed Libraries"=10, "Application Files"=11, "Boot Volume Root"=12] ("system directory type")
        w517 = "_"
        n164 = Unbundle By Name(w539) -> ("TrigCluster.TrigSource"=w511:T3, "HeaderString"=w513:string, "RecordedData"=w533:dbl[][])
        n165 = Array To Spreadsheet String(delimiter (Tab)=",", array=w533, 3:"%f" ("format string")) -> (spreadsheet string=w531:string)
        n166 = property on="TrigSource" class="Enum (strict)"(error in=w516) -> (error out=w515:errorcluster, "Strings []"=w514:string[])  [unwired: 1 in, 1 out]
        n167 = Index Array(array=w514, index=w511) -> (element=w512:string)
        n168 = Concatenate Strings(w513, "\r\n", "Time (s)", ",", "Speed (MPH)", "\r\n", w531) -> (w524:string)
        n169 = Get Date/Time In Seconds() -> (seconds since 1Jan1904=w528:timestamp)
        n170 = Format Date/Time String(time format string (%c)="%Y%m%d_%H%M%S", seconds (now)=w528) -> (date/time string=w519:string)  [unwired: 1 in]
        n171 = Concatenate Strings(w519, w517, w512, w517, w513, ".csv") -> (w526:string)
        n172 = call <vilib>:"Get System Directory.vi"("system directory type"=w530) -> ("system directory"=w529:path)  [unwired: 10 in]
        n173 = Build Path(base path=w529, name or relative path=w526) -> (appended path=w525:path)
        n174 = Write to Text File(file (use dialog)=w525, text=w524, error in=w515) -> (error out=w523:errorcluster)  [unwired: 1 in, 2 out]
      }
      frame "StreamingData" {
        w550 = FALSE  # Stop Loop?
        w551 = State."Restart"  # Next State
        w559 = T10 2 items=["User Home"=0, "User Desktop"=1, "User Documents"=2, "User Application Data"=3, "User Preferences"=4, "User Temporary"=5, "Public Documents"=6, "Public Application Data"=7, "Public Preferences"=8, "Public Cache"=13, "System Core Libraries"=9, "System Installed Libraries"=10, "Application Files"=11, "Boot Volume Root"=12] ("system directory type")
        w546 = "_"
        n175 = Unbundle By Name(w568) -> ("TrigCluster.TrigSource"=w540:T3, "HeaderString"=w542:string, "RecordedData"=w562:dbl[][])
        n176 = Array To Spreadsheet String(delimiter (Tab)=",", array=w562, 3:"%f" ("format string")) -> (spreadsheet string=w560:string)
        n177 = property on="TrigSource" class="Enum (strict)"(error in=w545) -> (error out=w544:errorcluster, "Strings []"=w543:string[])  [unwired: 1 in, 1 out]
        n178 = Index Array(array=w543, index=w540) -> (element=w541:string)
        n179 = Concatenate Strings(w542, "\r\n", "Time (s)", ",", "Speed (MPH)", "\r\n", w560) -> (w553:string)
        n180 = Get Date/Time In Seconds() -> (seconds since 1Jan1904=w557:timestamp)
        n181 = Format Date/Time String(time format string (%c)="%Y%m%d_%H%M%S", seconds (now)=w557) -> (date/time string=w548:string)  [unwired: 1 in]
        n182 = Concatenate Strings(w548, w546, w541, w546, w542, ".csv") -> (w555:string)
        n183 = call <vilib>:"Get System Directory.vi"("system directory type"=w559) -> ("system directory"=w558:path)  [unwired: 10 in]
        n184 = Build Path(base path=w558, name or relative path=w555) -> (appended path=w554:path)
        n185 = Write to Text File(file (use dialog)=w554, text=w553, error in=w544) -> (error out=w552:errorcluster)  [unwired: 1 in, 2 out]
      }
      frame "Restart" {
        w575 = State."Acquire"  # Next State
        w573 = 0.0 ("element")
        w577 = FALSE ("TriggerState")
        w579 = FALSE  # Stop Loop?
        n186 = Initialize Array(w573) -> (w572:dbl[])  [unwired: 1 in]
        n187 = Initialize Array(w573) -> (w574:dbl[][])  [unwired: 2 in]
        n188 = Bundle By Name(cluster=w580, "TriggerState"=w577, "PreTrigState"=w577, "StopButtonState"=w577, "Recording"=w577, "PreTrigStateCount"=u32 0, "RecordedData"=w574, "TrigTimeStamp"=w572) -> (w578:T6)
        n189 = property on="TrigSource" class="Enum (strict)"(error in=w571, "DisabledEnum"=T8."Enabled" ("Disabled")) -> (error out=w569:errorcluster)  [unwired: 1 in, 1 out]
      }
      frame "Exit" {
        w584 = TRUE  # Stop Loop?
        # "Exit - Exit the application."
      }
      frame "CheckPreTrigStateOrg" {
        w592 = FALSE  # Stop Loop?
        # "If PreTrigState True and TriggerState True then (Save MPH/Time Data).  If TriggerState False then check to see if the current speed is => min PreTrigState, if True then (Acquire) else Clear PreTrigState then (Acquire)"
        n190 = Unbundle By Name(w591) -> ("PreTrigState"=w595:bool, "Speed Data"=w589:dbl, "TrigSpeeds.StartSpeed"=w590:sgl)
        n191 = To Single Precision Float(number=w590) -> (single precision float=w588:sgl)
        n192 = call "CheckSpeedTol (SubVI).vi"("error in (no error)"=w587, "Target Speed"=w588, "Actual Speed"=w589) -> ("error out (no error)"=w586:errorcluster, "Speed in Range?"=w585:bool)  [unwired: 7 in]
        n193 = case shown="True" w595 {
          tunnel: w591 -> [w603 w624]
          tunnel: [w598 w626] -> w594
          tunnel: [w597 w625] -> w593
          tunnel: w585 -> [w596 w622]
          frame False {
            w597 = State."Acquire"  # Next State
            # "If the previous PreTrigState was false then check to see if the current belt speed meets the minimum speed for a PreTrigState."
            n194 = case shown="True" w596 {
              tunnel: w603 -> [w611 w618]
              tunnel: [w610 w617] -> w599
              frame False {
                # "Clears the PreTrigState and  timer value if the PreTrigState drops below 0.5 MPH"
                n195 = Bundle By Name(cluster=w611, "PreTrigState"=FALSE, "PreTrigTimer(s)"=0.0) -> (w610:T6)
              }
              frame True {
                # "Add currentMillisecondTimerValue to the Previous PreTrigTimer count and then if PreTrigTimer => 1.5 set PreTrigState True then (Acquire) eles (Acquire)"
                n196 = Unbundle By Name(w618) -> ("PreTrigTimer(s)"=w620:dbl, "MillisecondTimerValue"=w619:dbl)
                n197 = Tick Count (ms)() -> (millisecond timer value=w613:u32)
                n198 = To Double Precision Float(number=w613) -> (double precision float=w612:dbl)
                n199 = Subtract(x=w612, y=w619) -> (x-y=w621:dbl)
                n200 = Divide(x=w621, y=1000.0) -> (x/y=w616:dbl)
                n201 = Add(x=w620, y=w616) -> (x+y=w614:dbl)
                n202 = Bundle By Name(cluster=w618, "PreTrigTimer(s)"=w614) -> (w617:T6)
              }
            }
            n203 = Unbundle By Name(w599) -> ("PreTrigTimer(s)"=w602:dbl)
            n204 = Greater Or Equal?(x=w602, y=1.5) -> (x >= y?=w600:bool)
            n205 = case shown="True" w600 {
              tunnel: w599 -> [w604 w607]
              tunnel: [w604 w606] -> w598
              frame False {
              }
              frame True {
                n206 = Bundle By Name(cluster=w607, "PreTrigState"=TRUE) -> (w606:T6)
              }
            }
          }
          frame True {
            # "If TriggerState True then (Save MPH/Time Data)"
            n207 = Unbundle By Name(w624) -> ("TriggerState"=w623:bool)
            n208 = case shown="False" w623 {
              tunnel: [w629 w636] -> w626
              tunnel: w624 -> [w630 w636]
              tunnel: [w628 w635] -> w625
              tunnel: w622 -> [w627 _]
              frame False {
                w628 = State."Acquire"  # Next State
                # "If Speed Data is >= 0.5 then (Acquire) else clear PreTrigState then (Acqire)"
                n209 = case shown="False" w627 {
                  tunnel: w630 -> [w632 w634]
                  tunnel: [w631 w634] -> w629
                  frame False {
                    n210 = Bundle By Name(cluster=w632, "PreTrigState"=FALSE) -> (w631:T6)
                  }
                  frame True {
                  }
                }
              }
              frame True {
                w635 = State."Save MPH/Time Data"  # Next State
              }
            }
          }
        }
      }
      frame "Check TriggerOrg" {
        w641 = FALSE  # Stop Loop?
        w642 = State."Check for User Event"  # Next State
        # "If PreTrigState & NOT TriggerState is True, Then check TriggerLevel Data for a valid trigger and update TriggerState else do nothing."
        n211 = Unbundle By Name(w645) -> ("TriggerLevel Data"=w644:waveform(dbl)[], "PreTrigState"=w638:bool, "TriggerState"=w640:bool)  [unwired: 1 out]
        n212 = Not(x=w640) -> (.not. x?=w639:bool)
        n213 = And(x=w638, y=w639) -> (x .and. y?=w637:bool)
        n214 = case shown="True" w637 {
          tunnel: w645 -> [w647 w656]
          tunnel: w644 -> [_ w654]
          tunnel: [w647 w653] -> w643
          frame False {
          }
          frame True {
            n215 = Array Size(array=w654) -> (size(s)=w655:i32)
            n216 = for {
              N: w655 -> [_]
              tunnel: w654 -> [w664]
              tunnel: [w658] -> w652 mode=indexing
              i -> [w663]
              n217 = Index Array(array=w664, index=w663) -> (element=w662:waveform(dbl))
              n218 = Unbundle By Name(w662) -> ("Y"=w661:dbl[])
              n219 = Array Max & Min(array=w661) -> (max value=w660:dbl)  [unwired: 3 out]
              n220 = case shown="True" FALSE {
                tunnel: w660 -> [w667 w670]
                tunnel: 3.0 ("y") -> [w666 w669]
                tunnel: [w665 w668] -> w658
                frame False {
                  # "Checks for a Low Trigger State"
                  n221 = Less?(x=w667, y=w666) -> (x < y?=w665:bool)
                }
                frame True {
                  # "Checks for a High Trigger State"
                  n222 = Greater?(x=w670, y=w669) -> (0:w668:bool)
                }
              }
            }
            n223 = Search 1D Array(1D array=w652, element=TRUE) -> (index of element=w650:i32)  [unwired: 1 in]
            n224 = Not Equal?(x=w650, y=-1) -> (x != y?=w648:bool)
            n225 = Bundle By Name(cluster=w656, "TriggerState"=w648) -> (w653:T6)
          }
        }
      }
    }
    n226 = Equal?(x=w27, y=w28) -> (x = y?=w26:bool)
    n227 = case shown="True" w26 {
      tunnel: [w39 w40] -> w24
      tunnel: w25 -> [w39 _]
      frame False {
      }
      frame True {
        n228 = Tick Count (ms)() -> (millisecond timer value=w40:u32)
      }
    }
    n229 = Equal?(x=w31, y=w30) -> (x = y?=w29:bool)
    n230 = case shown="True" w29 {
      tunnel: w24 -> [w41 w44]
      tunnel: [w41 w42] -> w23
      frame False {
      }
      frame True {
        n231 = Tick Count (ms)() -> (millisecond timer value=w42:u32)
        n232 = Subtract(x=w42, y=w44) -> (x-y=→"Loop Time":u32)
      }
    }
    n233 = Or(x=w33, y=w35) -> (x .or. y?=w34:bool)
  }
  n234 = while {
    tunnel: w5 -> [w677]
    shift-right: [w672] -> w3
    shift-left: w14 -> [w673]
    stop <- w674 stop-if-true
    n235 = Dequeue Element(queue=w677, error in (no error)=w673) -> (queue out=w675:refnum<queue>, element=w676:T5, error out=w678:errorcluster)  [unwired: 1 in, 1 out]
    n236 = Unbundle By Name(w676) -> ("Message"=w680:enum16{"Init", "StopRFQ", "Stop", "UserEvent"}, "Message Data"=w679:variant)
    n237 = case shown="\"StopRFQ\"" w680 {
      tunnel: w679 -> [_ w691]
      tunnel: w678 -> [w682 w689]
      tunnel: w675 -> [_ w686]
      tunnel: [w682 w684] -> w672
      tunnel: [FALSE w683] -> w671
      frame "Init", Default {
      }
      frame "StopRFQ" {
        n238 = Variant To Data(error in=w689, type="", Variant=w691) -> (data=w688:string, error out=w685:errorcluster)
        n239 = Two Button Dialog(message=w688) -> (T button?=w687:bool)  [unwired: 2 in]
        n240 = case shown="False" w687 {
          tunnel: w686 -> [_ _]
          tunnel: w685 -> [w693 w695]
          tunnel: [w693 w695] -> w684
          tunnel: [FALSE TRUE] -> w683
          frame False {
          }
          frame True {
          }
        }
      }
    }
    "StopButton" <- w671
    n241 = Or(x=w671, y=w672) -> (x .or. y?=w674:bool)
  }
  n242 = Unbundle By Name(w7) -> ("AnalogTrigTask"=w10:refnum<k21>, "SpeedTask"=w9:refnum<k21>)
  n243 = call <vilib>:"DAQmx Clear Task.vi"("task in"=w9, "error in"=w6) -> ("error out"=w8:errorcluster)  [unwired: 13 in]
  n244 = call <vilib>:"DAQmx Clear Task.vi"("task in"=w10, "error in"=w8) -> ("error out"=w13:errorcluster)  [unwired: 13 in]
  n245 = Flush Queue(queue=w5, error in (no error)=w13) -> (queue out=w11:refnum<queue>, error out=w12:errorcluster)  [unwired: 1 out]
  n246 = Release Queue(queue=w11, error in (no error)=w12) -> (error out=w2:errorcluster)  [unwired: 1 in, 2 out]
  n247 = Merge Errors(w2, w3) -> (w4:errorcluster)
  n248 = call <vilib>:"Simple Error Handler.vi"("error in (no error)"=w4) -> ("error out"=w21:errorcluster)  [unwired: 4 in, 4 out]
  n249 = disable-structure shown="Default" {
    disable-tunnel: w21 -> [_ _]
    frame condition #0 (active) {
    }
    frame condition #1 {
      # "Call Quit LabVIEW if running as a built application."
      n250 = Quit LabVIEW() -> ()  [unwired: 1 in]
    }
  }
